vi "Dispose.vi"(8 "error in (no error)":errorcluster, 11 "ByRef":refnum<class "EnchantedMazeGame.lvclass">) -> (0 "error out":errorcluster)   [LabVIEW 2020, in "FactoryMethod.lvlib" / "NoParametrizedFactoryMethod.lvlib" / "EnchantedMazeGame.lvclass"]
uses:
  EnchantedMazeGame.lvclass
  EnchantedMazeGame.lvclass/EnchantedMazeGame.ctl
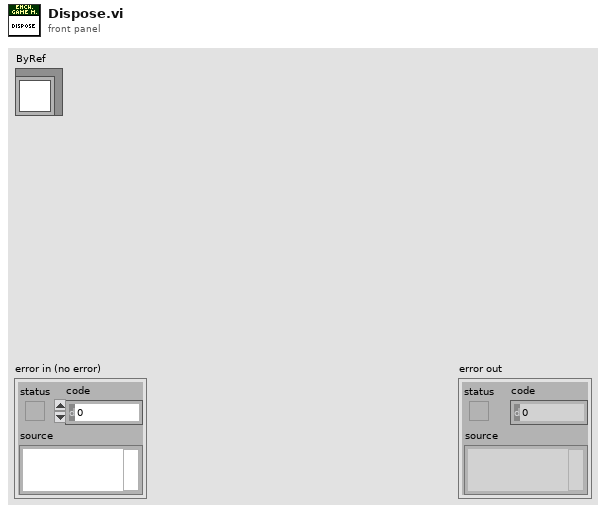
[diagram p1: front panel]
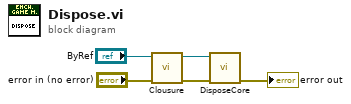
[diagram p0: block diagram]
diagram:
  n1 = call-dynamic "Clousure.vi"("error in (no error)"="error in (no error)", "MazeGame"="ByRef") -> ("error out"=w1:errorcluster, "MazeGame"=w2:refnum<class "EnchantedMazeGame.lvclass">)  [unwired: 8 in]
  n2 = call-dynamic "DisposeCore.vi"("error in (no error)"=w1, "MazeGame"=w2) -> ("error out"=→"error out":errorcluster)  [unwired: 8 in, 1 out]
